vi "Lorentzian2.vi"(3 "output control":T1, 4 "data":T2, 5 "X":dbl[](array[numeric]), 6 "a":dbl[](array[numeric])) -> (0 "error out":errorcluster, 1 "f'(X,a)":dbl[][](array[numeric]), 2 "f(X,a)":dbl[](array[numeric]))   [LabVIEW 2010]
doc: "This template is the starting point for creating a model function to be passed to the Nonlinear Curve Fit.vi."
uses:
  <vilib>/gmath/NumericalOptimization/objective function data.ctl
  <vilib>/gmath/NumericalOptimization/LM_output select.ctl
  <vilib>/gmath/NI_Gmath.lvlib
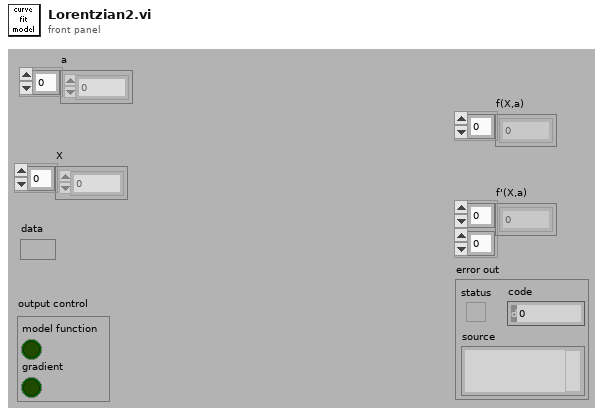
[diagram p1: front panel]
types:
  T1 = typedef "NI_Gmath.lvlib/LM_output select.ctl" = cluster{"model function":bool, "gradient":bool}
  T2 = typedef "NI_Gmath.lvlib/objective function data.ctl" = variant
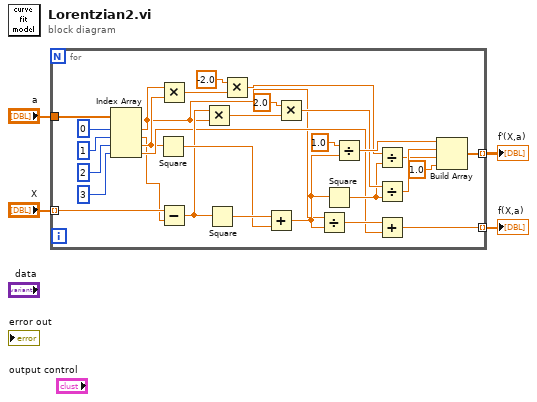
[diagram p0: block diagram]
diagram:
  n1 = for {
    tunnel: "a" -> [w33]
    tunnel: "X" -> [w11] mode=indexing
    tunnel: [w15] -> w2 mode=indexing
    tunnel: [w14] -> w1 mode=indexing
    n2 = Index Array(array=w33, index #1=0 ("index"), index #2=1 ("index"), index #3=2 ("index"), index #4=3 ("index")) -> (element #1=w6:dbl, element #2=w5:dbl, element #3=w12:dbl, element #4=w13:dbl)
    n3 = Square(x=w12) -> (x^2=w30:dbl)
    n4 = Multiply(x=w6, y=w12) -> (x*y=w19:dbl)
    n5 = Subtract(x=w11, y=w5) -> (x-y=w24:dbl)
    n6 = Multiply(x=w24, y=w6) -> (x*y=w25:dbl)
    n7 = Square(x=w24) -> (x^2=w31:dbl)
    n8 = Multiply(x=-2.0, y=w19) -> (x*y=w18:dbl)
    n9 = Add(x=w31, y=w30) -> (x+y=w22:dbl)
    n10 = Multiply(x=2.0, y=w25) -> (x*y=w23:dbl)
    n11 = Divide(x=w6, y=w22) -> (x/y=w29:dbl)
    n12 = Square(x=w22) -> (x^2=w17:dbl)
    n13 = Divide(x=1.0, y=w22) -> (x/y=w27:dbl)
    n14 = Divide(x=w18, y=w17) -> (x/y=w16:dbl)
    n15 = Divide(x=w23, y=w17) -> (x/y=w21:dbl)
    n16 = Add(x=w29, y=w13) -> (x+y=w14:dbl)
    n17 = Build Array(w27, w21, w16, 1.0) -> (w15:dbl[])
  }
  "f(X,a)" <- w1
  "f'(X,a)" <- w2
